vi "WriteCompressed_Digitizer.vi"(5 "Module":string="data", 7 "name":string, 8 "error in":errorcluster, 10 "data":u16[][](array[numeric])=[[1, 2, 3, 4], [9, 8, 7, 6], [100, 200, 300, 400]], 11 "File Handle":T1 format="%.0x") -> (0 "error out":errorcluster)   [LabVIEW 2014]
uses:
  <vilib>/addons/h5labview2/base/hid_t.ctl
  <vilib>/addons/h5labview2/base/lib_path.vi
  <vilib>/addons/h5labview2/base/H5Equery.vi
  <vilib>/addons/h5labview2/dataset/H5Dwrite.llb/H5Dwrite.xnode
  <vilib>/addons/h5labview2/space/H5S.lvlib
  <vilib>/addons/h5labview2/dataset/H5D.lvlib
  <vilib>/addons/h5labview2/type/H5T.lvlib
  <vilib>/addons/h5labview2/props/H5P.lvlib
  <vilib>/addons/h5labview2/group/H5G.lvlib
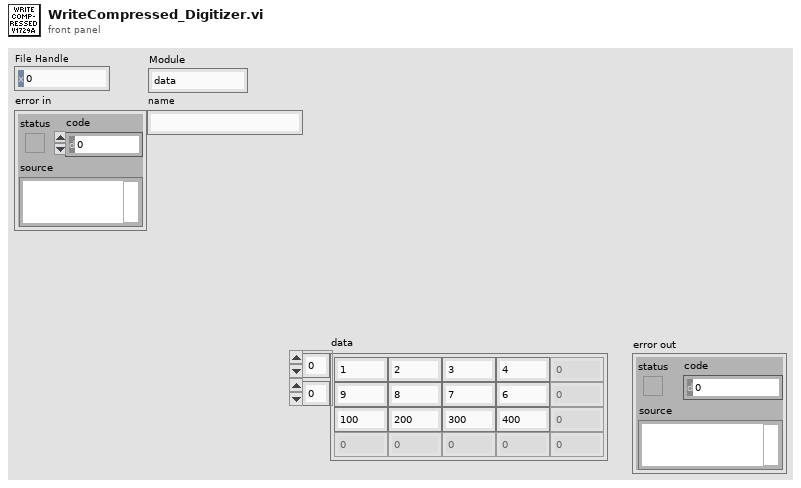
[diagram p1: front panel]
types:
  T1 = typedef "hid_t.ctl" = i32
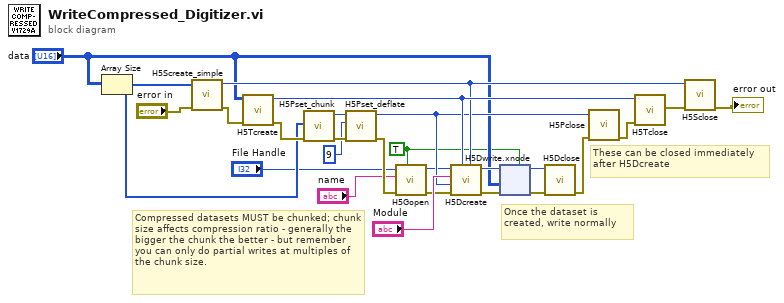
[diagram p0: block diagram]
diagram:
  w2 = TRUE ("create? (F)")
  # "Once the dataset is created, write normally"
  # "Compressed datasets MUST be chunked; chunk size affects compression ratio - generally the bigger the chunk the better - but remember you can only do partial writes at multiples of the chunk size."
  # "These can be closed immediately after H5Dcreate"
  n1 = Array Size(array="data") -> (size(s)=w8:i32[])
  n2 = call <vilib>:"H5Screate_simple.vi"("error in (no error)"="error in", "dims"=w8) -> ("error out"=w26:errorcluster, "space out"=w19:T1)  [unwired: 7 in, 1 out]
  n3 = call <vilib>:"H5Tcreate.vi"("error in (no error)"=w26, "type variant"="data") -> ("error out"=w14:errorcluster, "type out"=w20:i32)  [unwired: 7 in, 1 out]
  n4 = call <vilib>:"H5Pset_chunk.vi"("error in (no error)"=w14, "chunk size"=w8) -> ("error out"=w13:errorcluster, "prop out"=w12:T1)  [unwired: 8 in]
  n5 = call <vilib>:"H5Pset_deflate.vi"("error in (no error)"=w13, "level"=u8 9, "prop in"=w12) -> ("error out"=w6:errorcluster, "prop out"=w16:T1)  [unwired: 7 in]
  n6 = call <vilib>:"H5Gopen.vi"("create? (F)"=w2, "error in (no error)"=w6, "name"="name", "ref in"="File Handle") -> ("error out"=w5:errorcluster, "group out"=w1:T1)  [unwired: 6 in]
  n7 = call <vilib>:"H5Dcreate.vi"("space id"=w19, "type id"=w20, "error in (no error)"=w5, "props id"=w16, "name"="Module", "loc in"=w1) -> ("error out"=w24:errorcluster, "dset out"=w23:T1)  [unwired: 2 in]
  n8 = xnode "H5Dwrite.xnode"("replace? (F)"=w2, "error in (no error)"=w24, "data"="data", "ref in"=w23) -> ("error out"=w22:errorcluster, "ref out"=w21:T1)  [unwired: 3 in, 1 out]
  n9 = call <vilib>:"H5Dclose.vi"("error in (no error)"=w22, "dset in"=w21) -> ("error out"=w7:errorcluster)  [unwired: 9 in]
  n10 = call <vilib>:"H5Pclose.vi"("error in (no error)"=w7, "props in"=w16) -> ("error out"=w17:errorcluster)  [unwired: 9 in]
  n11 = call <vilib>:"H5Tclose.vi"("error in (no error)"=w17, "type in"=w20) -> ("error out"=w18:errorcluster)  [unwired: 9 in]
  n12 = call <vilib>:"H5Sclose.vi"("error in (no error)"=w18, "space in"=w19) -> ("error out"=→"error out":errorcluster)  [unwired: 9 in]
